vi "Test Parameter and Results.vi"() -> ()   [LabVIEW 2020, in "XML Handler.lvclass"]
uses:
  XML Handler.lvclass
  Devices/Controls/Device Information Cluster.ctl
  Devices/Controls/Register to Write.ctl
  Controls/Result Cluster.ctl
  XML Handler.lvclass/XML Handler.ctl
  Measurements/Support VI/Update parameters (array).vi
  <resource>/objmgr/DOMUserDefRef.rc
  Measurements/Measurement.lvclass
  Devices/PIC-device/PIC-Device.lvclass
  Devices/Device.lvclass
  Test Framework/Test Framework.lvclass
panel:
  in  "PSUs in parameters":bool
  in  "Parameter names":string[][](array[string])
  out "error out":errorcluster
  in  "Output File Folder":path=path "C:/Users/niko.kuusniemi/Documents/temp/Framework temp/test.xml"
  out "Numeric Control":i32
  out "XML":string
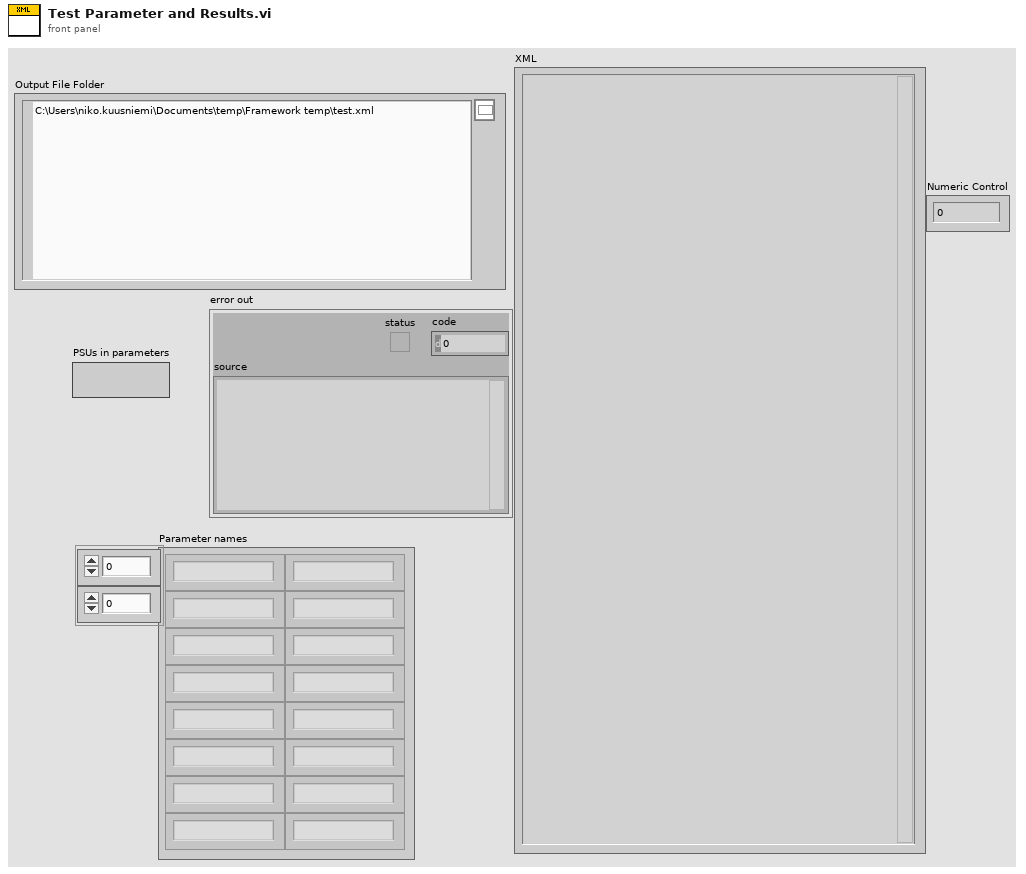
[diagram p1: front panel]
types:
  T1 = typedef "Device.lvclass/Device Information Cluster.ctl" = cluster{"Device Info":string[][], "Default Values":T2[], "Fetched info":string[][]}
  T2 = typedef "PIC-Device.lvclass/Register to Write.ctl" = cluster{"Register":u32, "Value":u32, "Dev Address":u32, "Physical Adress":u32}
  T3 = cluster{"Temperature [degC]":dbl, "Soak time [s]":dbl, "PSUs":cluster{"PSU alias":string, "Source":enum32{"Voltage", "Current"}, "Drive (V/A)":dbl}[]}
  T4 = cluster{"PSU alias":string, "Source":enum32{"Voltage", "Current"}, "Drive (V/A)":dbl}[]
  T5 = cluster{"Temperature [degC]":dbl, "Soak time [s]":dbl, "PSUs":cluster{"PSU alias":string, "Source":enum32{"Voltage", "Current"}, "Drive (V/A)":dbl}[]}[]
  T6 = typedef "XML Handler.lvclass/Result Cluster.ctl" = cluster{"Name":string, "Value":string}
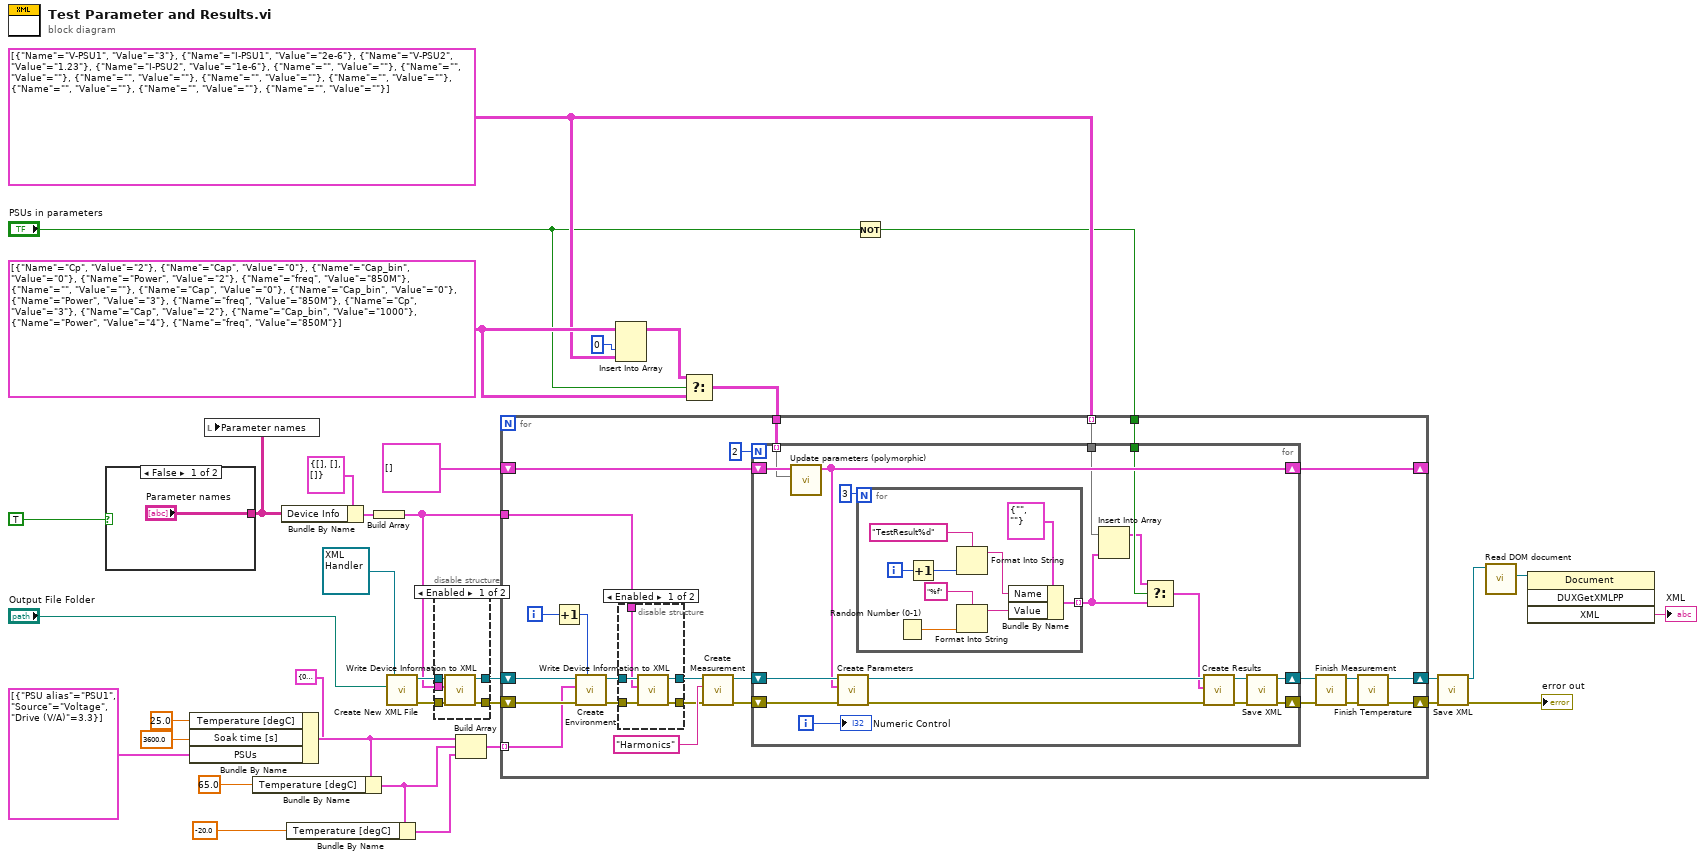
[diagram p0: block diagram]
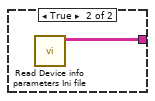
[diagram p3: hidden frame]
diagram:
  w4 = cluster{"Name":string, "Value":string}[][] [[{"Name"="V-PSU1", "Value"="3"}, {"Name"="I-PSU1", "Value"="2e-6"}, {"Name"="V-PSU2", "Value"="1.23"}, {"Name"="I-PSU2", "Value"="1e-6"}], [{"Name"="", "Value"=""}, {"Name"="", "Value"=""}, {"Name"="", "Value"=""}, {"Name"="", "Value"=""}], [{"Name"="", "Value"=""}, {"Name"="", "Value"=""}, {"Name"="", "Value"=""}, {"Name"="", "Value"=""}]] ("Parameters")
  w7 = cluster{"Name":string, "Value":string}[][] [[{"Name"="Cp", "Value"="2"}, {"Name"="Cap", "Value"="0"}, {"Name"="Cap_bin", "Value"="0"}, {"Name"="Power", "Value"="2"}, {"Name"="freq", "Value"="850M"}], [{"Name"="", "Value"=""}, {"Name"="Cap", "Value"="0"}, {"Name"="Cap_bin", "Value"="0"}, {"Name"="Power", "Value"="3"}, {"Name"="freq", "Value"="850M"}], [{"Name"="Cp", "Value"="3"}, {"Name"="Cap", "Value"="2"}, {"Name"="Cap_bin", "Value"="1000"}, {"Name"="Power", "Value"="4"}, {"Name"="freq", "Value"="850M"}]] ("Parameters")
  n1 = case shown="False" TRUE {
    tunnel: ["Parameter names" w37] -> w9
    frame False {
    }
    frame True {
      n2 = call "Read Device info parameters Ini file.vi"() -> ("Instrument info"=w37:string[][])  [unwired: 8 in, 3 out]
    }
  }
  n3 = Bundle By Name(cluster=T3 {"Temperature [degC]"=0.0, "Soak time [s]"=0.0, "PSUs"=[]} ("Environmental info"), "Temperature [degC]"=25.0, "Soak time [s]"=3600.0, "PSUs"=T4 [{"PSU alias"="PSU1", "Source"=enum."Voltage", "Drive (V/A)"=3.3}]) -> (w28:T3)
  n4 = local write "Parameter names"(w9) -> ()
  n5 = Bundle By Name(cluster=w28, "Temperature [degC]"=65.0) -> (w26:T3)
  n6 = Bundle By Name(cluster=T1 {"Device Info"=[], "Default Values"=[], "Fetched info"=[]} ("Device Defaults"), "Device Info"=w9) -> (w11:T1)
  n7 = Bundle By Name(cluster=w26, "Temperature [degC]"=-20.0) -> (w27:T3)
  n8 = Build Array(w11) -> (w1:T1[])
  n9 = call "Create New XML File.vi"("Output File Folder"="Output File Folder", "XML Handler in"=refnum<class "XML Handler.lvclass"> refnum) -> ("error out"=w16:errorcluster, "XML Handler out"=w15:refnum<class "XML Handler.lvclass">)  [unwired: 8 in]
  n10 = disable-structure shown="Enabled" {
    disable-tunnel: w16 -> [w42 w44]
    disable-tunnel: w15 -> [w41 w43]
    disable-tunnel: [w40 w44] -> w14
    disable-tunnel: [w39 w43] -> w13
    disable-tunnel: w1 -> [w38 _]
    frame Enabled {
      n11 = call "Write Device Information to XML.vi"("error in (no error)"=w42, "Device Information"=w38, "XML Handler in"=w41) -> ("error out"=w40:errorcluster, "XML Handler out"=w39:refnum<class "XML Handler.lvclass">)  [unwired: 7 in]
    }
    frame Disabled {
    }
  }
  n12 = Build Array(w28, w26, w27) -> (w25:T5)
  n13 = Insert Into Array(array=w7, index (col)=0 ("disabled index (col)"), new element=w4) -> (w8:cluster{"Name":string, "Value":string}[][])  [unwired: 1 in]
  n14 = Select(t=w8, s="PSUs in parameters", f=w7) -> (s? t:f=w6:cluster{"Name":string, "Value":string}[][])
  n15 = Not(x="PSUs in parameters") -> (.not. x?=w2:bool)
  n16 = for {
    shift-right: [w59] -> w20
    shift-left: w14 -> [w64]
    shift-right: [w60] -> w18
    shift-left: w13 -> [w61]
    tunnel: w25 -> [w58] mode=indexing
    shift-right: [w57] -> _
    shift-left: cluster{"Name":string, "Value":string}[] [] ("Parameters") -> [w53]
    tunnel: w6 -> [w52]
    tunnel: w4 -> [w51] mode=indexing
    tunnel: w2 -> [w50]
    tunnel: w1 -> [w45]
    i -> [w55]
    n17 = Increment(x=w55) -> (x+1=w54:i32)
    n18 = call "Create Environment.vi"("Environmental index"=w54, "error in (no error)"=w64, "Environmental info"=w58, "XML Handler in"=w61) -> ("error out"=w48:errorcluster, "XML Handler out"=w49:refnum<class "XML Handler.lvclass">)  [unwired: 6 in]
    n19 = disable-structure shown="Enabled" {
      disable-tunnel: w49 -> [w74 w76]
      disable-tunnel: w48 -> [w73 w75]
      disable-tunnel: [w72 w76] -> w47
      disable-tunnel: [w71 w75] -> w46
      disable-tunnel: w45 -> [w70 _]
      frame Enabled {
        n20 = call "Write Device Information to XML.vi"("error in (no error)"=w73, "Device Information"=w70, "XML Handler in"=w74) -> ("error out"=w71:errorcluster, "XML Handler out"=w72:refnum<class "XML Handler.lvclass">)  [unwired: 7 in]
      }
      frame Disabled {
      }
    }
    n21 = call "Create Measurement.vi"("error in (no error)"=w46, "Measurement Name"="Harmonics", "XML Handler in"=w47) -> ("error out"=w68:errorcluster, "XML Handler out"=w67:refnum<class "XML Handler.lvclass">)  [unwired: 7 in]
    n22 = for {
      N: 2 -> [_]
      shift-right: [w84] -> w65
      shift-left: w68 -> [w94]
      shift-right: [w83] -> w66
      shift-left: w67 -> [w93]
      shift-right: [w88] -> w57
      shift-left: w53 -> [w89]
      tunnel: w52 -> [w82] mode=indexing
      tunnel: w51 -> [w81]
      tunnel: w50 -> [w80]
      i -> [w87]
      n23 = call-poly "Update parameters (polymorphic).vi"("New Parameters"=w82, "Parameters"=w89) -> ("Parameters Out"=w88:cluster{"Name":string, "Value":string}[])  [unwired: 9 in]
      n24 = call "Create Parameters.vi"("error in (no error)"=w94, "Parameters"=w88, "XML Handler in"=w93) -> ("error out"=w91:errorcluster, "XML Handler out"=w92:refnum<class "XML Handler.lvclass">)  [unwired: 7 in]
      n25 = for {
        N: 3 -> [_]
        tunnel: [w100] -> w78 mode=indexing
        i -> [w102]
        n26 = Random Number (0-1)() -> (number: 0 to 1=w96:dbl)
        n27 = Increment(x=w102) -> (x+1=w101:i32)
        n28 = Format Into String(format string="TestResult%d" ("Name"), w101) -> (resulting string=w98:string)  [unwired: 2 in, 1 out]
        n29 = Format Into String(format string="%f" ("Name"), w96) -> (resulting string=w97:string)  [unwired: 2 in, 1 out]
        n30 = Bundle By Name(cluster=T6 {"Name"="", "Value"=""} ("Result Cluster"), "Name"=w98, "Value"=w97) -> (w100:T6)
      }
      n31 = Insert Into Array(array=w81, new element=w78) -> (w79:cluster{"Name":string, "Value":string}[])  [unwired: 1 in]
      n32 = Select(t=w79, s=w80, f=w78) -> (s? t:f=w77:T6[])
      n33 = call "Create Results.vi"("error in (no error)"=w91, "Results"=w77, "XML Handler in"=w92) -> ("error out"=w85:errorcluster, "XML Handler out"=w86:refnum<class "XML Handler.lvclass">)  [unwired: 7 in]
      n34 = call "Save XML.vi"("error in (no error)"=w85, "XML Handler in"=w86) -> ("error out"=w84:errorcluster, "XML Handler out"=w83:refnum<class "XML Handler.lvclass">)  [unwired: 8 in]
      "Numeric Control" <- w87
    }
    n35 = call-dynamic "Finish Measurement.vi"("error in (no error)"=w65, "XML Handler in"=w66) -> ("error out"=w63:errorcluster, "XML Handler out"=w62:refnum<class "XML Handler.lvclass">)  [unwired: 8 in]
    n36 = call "Finish Temperature.vi"("error in (no error)"=w63, "XML Handler in"=w62) -> ("error out"=w59:errorcluster, "XML Handler out"=w60:refnum<class "XML Handler.lvclass">)  [unwired: 8 in]
  }
  n37 = call "Save XML.vi"("error in (no error)"=w20, "XML Handler in"=w18) -> ("error out"=→"error out":errorcluster, "XML Handler out"=w17:refnum<class "XML Handler.lvclass">)  [unwired: 8 in]
  n38 = call "Read DOM document.vi"("XML Handler in"=w17) -> ("DOM document"=w35:refnum<k20>)  [unwired: 9 in, 1 out]
  n39 = invoke class="Document" method="DUXGetXMLPP"(reference=w35) -> ("XML"=→"XML":string)  [unwired: 3 in, 3 out]
